vi "Victory Message.vi"(11 "MyTeam":refnum<class "MyTeam.lvclass">) -> (2 "Victory Message":string)   [LabVIEW 2020, in "Clones.lvlib" / "MyTeam.lvclass"]
uses:
  MyTeam.lvclass
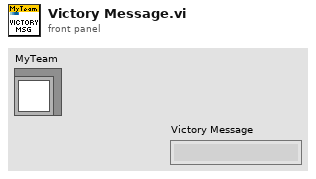
[diagram p1: front panel]
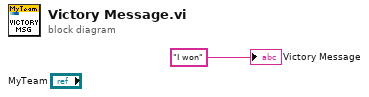
[diagram p0: block diagram]
diagram:
  "Victory Message" <- "I won" ("Victory Message")
